vi "TLPM_OpenCloseConn.vi"(7 "Open":bool, 8 "error in":errorcluster, 10 "Retry":bool, 11 "ConnID":refnum<visa-resource-name>) -> (0 "error out":errorcluster, 3 "connection ID":refnum<visa-resource-name>)   [LabVIEW 2019]
uses:
  <vilib>/Utility/config.llb/Read Key (U32).vi
  <vilib>/Utility/config.llb/Write Key (U32).vi
  <vilib>/Utility/config.llb/Read Key (String).vi
  <vilib>/Utility/config.llb/Read Key (I32).vi
  <vilib>/Utility/config.llb/Read Key (Boolean).vi
  <vilib>/Utility/config.llb/Write Key (String).vi
  <vilib>/Utility/config.llb/Write Key (Boolean).vi
  <vilib>/Utility/config.llb/Write Key (I32).vi
  <vilib>/Utility/config.llb/NI_LVConfig.lvlib
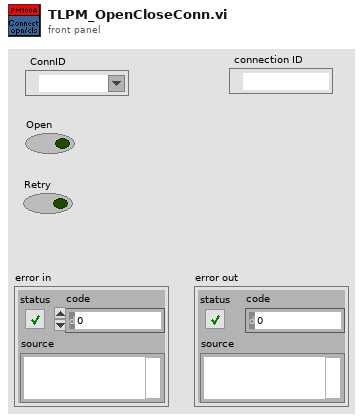
[diagram p1: front panel]
types:
  T1 = enum16{"Répertoire du VI actuel", "Répertoire du parent 1", "Répertoire du parent 2", "Répertoire du parent 3"}
  T2 = typedef "NI_LVConfig.lvlib/Config Data RefNum.ctl" = refnum<k1>
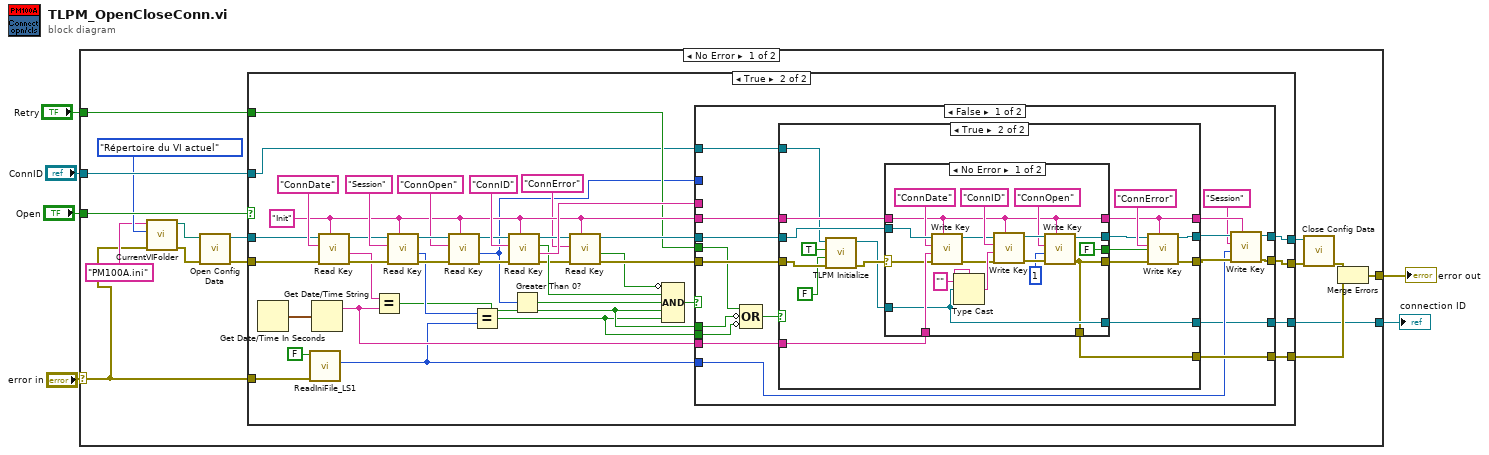
[diagram p0: block diagram]
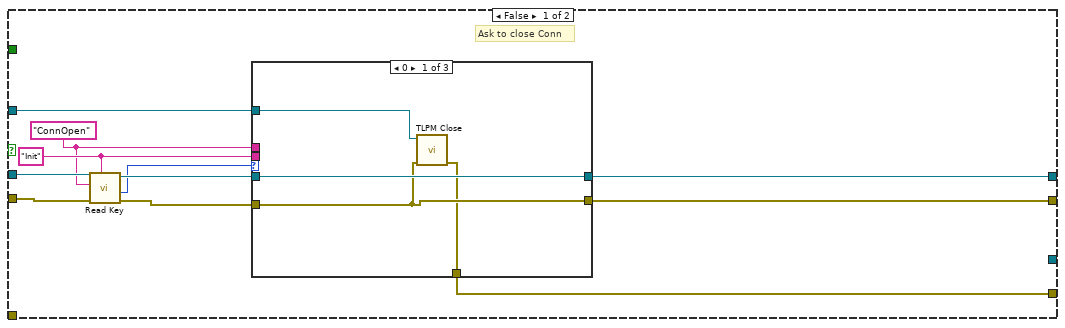
[diagram p2: hidden frame]
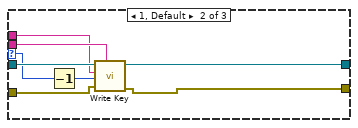
[diagram p3: hidden frame]
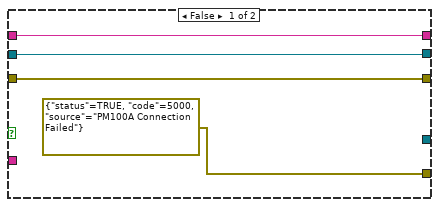
[diagram p5: hidden frame]
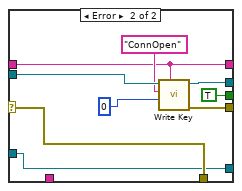
[diagram p6: hidden frame]
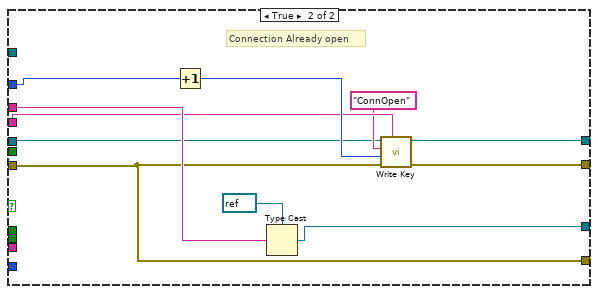
[diagram p7: hidden frame]
diagram:
  n1 = case shown="No Error" "error in" {
    selector: "error in" -> [w11 w166]
    tunnel: [w15 w166] -> w6
    tunnel: "Open" -> [w21 _]
    tunnel: [w7 w165] -> w4
    tunnel: "ConnID" -> [w22 w165]
    tunnel: "Retry" -> [w8 _]
    frame No Error {
      n2 = call <userlib>:"CurrentVIFolder.vi"("error in (no error)"=w11, "Source"=T1."Répertoire du VI actuel", "NomFichier"="PM100A.ini" ("nom ou chemin relatif")) -> ("error out"=w10:errorcluster, "Chemin"=w9:path)  [unwired: 6 in, 1 out]
      n3 = call <vilib>:"Open Config Data.vi"("error in (no error)"=w10, "configuration file path"=w9) -> ("error out"=w20:errorcluster, "refnum"=w19:T2)  [unwired: 7 in, 1 out]
      n4 = case shown="True" w21 {
        tunnel: w22 -> [w32 w48]
        tunnel: w11 -> [_ w80]
        tunnel: [w31 w72] -> w16
        tunnel: w20 -> [w30 w71]
        tunnel: w19 -> [w27 w70]
        tunnel: [w33 w63] -> w18
        tunnel: [w23 w62] -> w17
        tunnel: w8 -> [_ w52]
        tunnel: [_ w49] -> w7
        frame False {
          w28 = "Init" ("section")
          w25 = "ConnOpen" ("key")
          # "Ask to close Conn"
          n5 = call-poly <vilib>:"Read Key.vi"("section"=w28, "error in (no error)"=w30, "key"=w25, "refnum"=w27) -> ("error out"=w29:errorcluster, "value"=w24:u32, "refnum out"=w26:T2)  [unwired: 4 in, 1 out]
          n6 = case shown="0" w24 {
            selector: w24 -> [_ w38 _]
            tunnel: [w37 w45 w47] -> w33
            tunnel: w32 -> [w36 _ _]
            tunnel: [w34 _ w46] -> w31
            tunnel: w29 -> [w35 w44 w46]
            tunnel: w28 -> [_ w43 _]
            tunnel: w26 -> [w37 w42 w47]
            tunnel: w25 -> [_ w41 _]
            tunnel: [w35 w40 w46] -> w23
            frame 0 {
              n7 = call <userlib>:"TLPM Close.vi"("error in (no error)"=w35, "instrument handle"=w36) -> ("error out"=w34:errorcluster)  [unwired: 9 in]
            }
            frame 1, Default {
              n8 = Decrement(x=w38) -> (x-1=w39:u32)
              n9 = call-poly <vilib>:"Write Key.vi"("section"=w43, "error in (no error)"=w44, "value"=w39, "key"=w41, "refnum"=w42) -> ("error out"=w40:errorcluster, "refnum out"=w45:T2)  [unwired: 4 in, 1 out]
            }
            frame 2 {
            }
          }
        }
        frame True {
          w57 = "Init" ("section")
          n10 = Get Date/Time In Seconds() -> (seconds since 1Jan1904=w79:timestamp)
          n11 = call "ReadIniFile_LS1.vi"("Error in"=w80, "UpdateSess"=FALSE ("IncrSession")) -> ("Session"=w73:i32)  [unwired: 3 in, 6 out]
          n12 = Get Date/Time String(seconds (now)=w79) -> (date string=w74:string)  [unwired: 2 in, 1 out]
          n13 = call-poly <vilib>:"Read Key.vi"("section"=w57, "error in (no error)"=w71, "key"="ConnDate", "refnum"=w70) -> ("error out"=w84:errorcluster, "value"=w78:string, "refnum out"=w82:T2)  [unwired: 4 in, 1 out]
          n14 = Equal?(x=w78, y=w74) -> (x = y?=w56:bool)
          n15 = call-poly <vilib>:"Read Key.vi"("section"=w57, "error in (no error)"=w84, "key"="Session", "refnum"=w82) -> ("error out"=w69:errorcluster, "value"=w68:i32, "refnum out"=w67:T2)  [unwired: 4 in, 1 out]
          n16 = call-poly <vilib>:"Read Key.vi"("section"=w57, "error in (no error)"=w69, "key"="ConnOpen", "refnum"=w67) -> ("error out"=w65:errorcluster, "value"=w50:u32, "refnum out"=w64:T2)  [unwired: 4 in, 1 out]
          n17 = Equal?(x=w68, y=w73) -> (x = y?=w55:bool)
          n18 = call-poly <vilib>:"Read Key.vi"("section"=w57, "error in (no error)"=w65, "key"="ConnID", "refnum"=w64) -> ("error out"=w61:errorcluster, "value"=w77:string, "found?"=w76:bool, "refnum out"=w58:T2)  [unwired: 4 in]
          n19 = Greater Than 0?(x=w50) -> (x > 0?=w51:bool)
          n20 = call-poly <vilib>:"Read Key.vi"("section"=w57, "error in (no error)"=w61, "key"="ConnError", "refnum"=w58) -> ("error out"=w60:errorcluster, "value"=w53:bool, "refnum out"=w59:T2)  [unwired: 4 in, 1 out]
          n21 = Compound Arithmetic op=AND ("Opérateur arithmétique")(invert w53, w76, w51, w56, w55) -> (w75:bool)
          n22 = case shown="False" w75 {
            tunnel: w77 -> [_ w164]
            tunnel: w60 -> [w104 w163]
            tunnel: w59 -> [w103 w157]
            tunnel: w74 -> [w102 _]
            tunnel: w73 -> [w89 _]
            tunnel: w57 -> [w101 w160]
            tunnel: [w100 w163] -> w72
            tunnel: [w91 w156] -> w63
            tunnel: [w90 w158] -> w62
            tunnel: w56 -> [w97 _]
            tunnel: w55 -> [w96 _]
            tunnel: w52 -> [w99 _]
            tunnel: w50 -> [_ w162]
            tunnel: [w88 w154] -> w49
            tunnel: w48 -> [w87 _]
            frame False {
              n23 = Compound Arithmetic op=OR ("Opérateur arithmétique")(w99, invert w97, invert w96) -> (w98:bool)
              n24 = case shown="True" w98 {
                tunnel: w104 -> [w106 w114]
                tunnel: w103 -> [w108 w126]
                tunnel: w102 -> [_ w125]
                tunnel: w101 -> [w105 w124]
                tunnel: [_ w123] -> w88
                tunnel: [w108 w117] -> w95
                tunnel: [w106 w118] -> w94
                tunnel: [errorcluster {"status"=TRUE, "code"=5000, "source"="PM100A Connection Failed"} ("error IO") w122] -> w100
                tunnel: [w105 w115] -> w93
                tunnel: w87 -> [_ w111]
                frame False {
                }
                frame True {
                  n25 = call <userlib>:"TLPM Initialize.vi"("error in (no error)"=w114, "Reset Device (Reset Device)"=FALSE, "ID Query (Do Query)"=TRUE, "resource name"=w111) -> ("error out"=w113:errorcluster, "instrument handle out"=w112:refnum<visa-resource-name>)  [unwired: 6 in]
                  n26 = case shown="No Error" w113 {
                    selector: w113 -> [w138 w147]
                    tunnel: w126 -> [w144 w153]
                    tunnel: w125 -> [w142 _]
                    tunnel: w124 -> [w132 w149]
                    tunnel: w112 -> [w139 w145]
                    tunnel: [w139 w145] -> w123
                    tunnel: [w133 w152] -> w119
                    tunnel: [w134 w151] -> w120
                    tunnel: [w133 w147] -> w122
                    tunnel: [w132 w149] -> w115
                    tunnel: [FALSE ("value") TRUE ("value")] -> w116
                    frame No Error {
                      n27 = call-poly <vilib>:"Write Key.vi"("section"=w132, "error in (no error)"=w138, "value"=w142, "key"="ConnDate", "refnum"=w144) -> ("error out"=w129:errorcluster, "refnum out"=w130:T2)  [unwired: 4 in, 1 out]
                      n28 = Type Cast(type="", x=w139) -> (*(type *) &x=w141:string)
                      n29 = call-poly <vilib>:"Write Key.vi"("section"=w132, "error in (no error)"=w129, "value"=w141, "key"="ConnID", "refnum"=w130) -> ("error out"=w136:errorcluster, "refnum out"=w137:T2)  [unwired: 4 in, 1 out]
                      n30 = call-poly <vilib>:"Write Key.vi"("section"=w132, "error in (no error)"=w136, "value"=u32 1, "key"="ConnOpen", "refnum"=w137) -> ("error out"=w133:errorcluster, "refnum out"=w134:T2)  [unwired: 4 in, 1 out]
                    }
                    frame Error {
                      n31 = call-poly <vilib>:"Write Key.vi"("section"=w149, "value"=u32 0, "key"="ConnOpen", "refnum"=w153) -> ("error out"=w152:errorcluster, "refnum out"=w151:T2)  [unwired: 5 in, 1 out]
                    }
                  }
                  n32 = call-poly <vilib>:"Write Key.vi"("section"=w115, "error in (no error)"=w119, "value"=w116, "key"="ConnError", "refnum"=w120) -> ("error out"=w118:errorcluster, "refnum out"=w117:T2)  [unwired: 4 in, 1 out]
                }
              }
              n33 = call-poly <vilib>:"Write Key.vi"("section"=w93, "error in (no error)"=w94, "value"=w89, "key"="Session", "refnum"=w95) -> ("error out"=w90:errorcluster, "refnum out"=w91:T2)  [unwired: 4 in, 1 out]
            }
            frame True {
              # "Connection Already open"
              n34 = Increment(x=w162) -> (x+1=w161:u32)
              n35 = Type Cast(type=refnum<visa-resource-name> refnum ("VISA resource name"), x=w164) -> (*(type *) &x=w154:refnum<visa-resource-name>)
              n36 = call-poly <vilib>:"Write Key.vi"("section"=w160, "error in (no error)"=w163, "value"=w161, "key"="ConnOpen", "refnum"=w157) -> ("error out"=w158:errorcluster, "refnum out"=w156:T2)  [unwired: 4 in, 1 out]
            }
          }
        }
      }
      n37 = call <vilib>:"Close Config Data.vi"("error in (no error)"=w17, "refnum"=w18) -> ("error out"=w14:errorcluster)  [unwired: 8 in, 1 out]
      n38 = Merge Errors(w14, w16) -> (w15:errorcluster)
    }
    frame Error {
    }
  }
  "error out" <- w6
  "connection ID" <- w4
